vi "Table Test Sequencer.vi"(10 "Action":T1=enum."Run Position", 11 "Test Table":string[][](table)=[["1", "10mA", "10"], ["2", "20mA", "20"], ["3", "100mA", "10"], ["4", "20mA", "20"]]) -> (0 "Current Elapsed":dbl format="%.2g", 1 "CountDown Time":dbl format="%.2g", 2 "Test Running":bool, 3 "Current Test":string[](array[string]), 4 "Current Step ID":i32=-1, 5 "CountDown Pie":picture, 6 "Test Table Out":string[][](array[string])=[["1", "10mA", "1"], ["2", "20mA", "2"], ["3", "100mA", "1"], ["4", "20mA", "2"]], 7 "CountDown Text":string="0:00")   [LabVIEW 2018]
uses:
  Controls/StateMachineStates_TEST_TDEF.ctl
  Controls/Step Control Methods ENUM_TEST_TDef.ctl
  Controls/Timer Actions ENUM_TEST_TDef.ctl
  Controls/Stability State.ctl
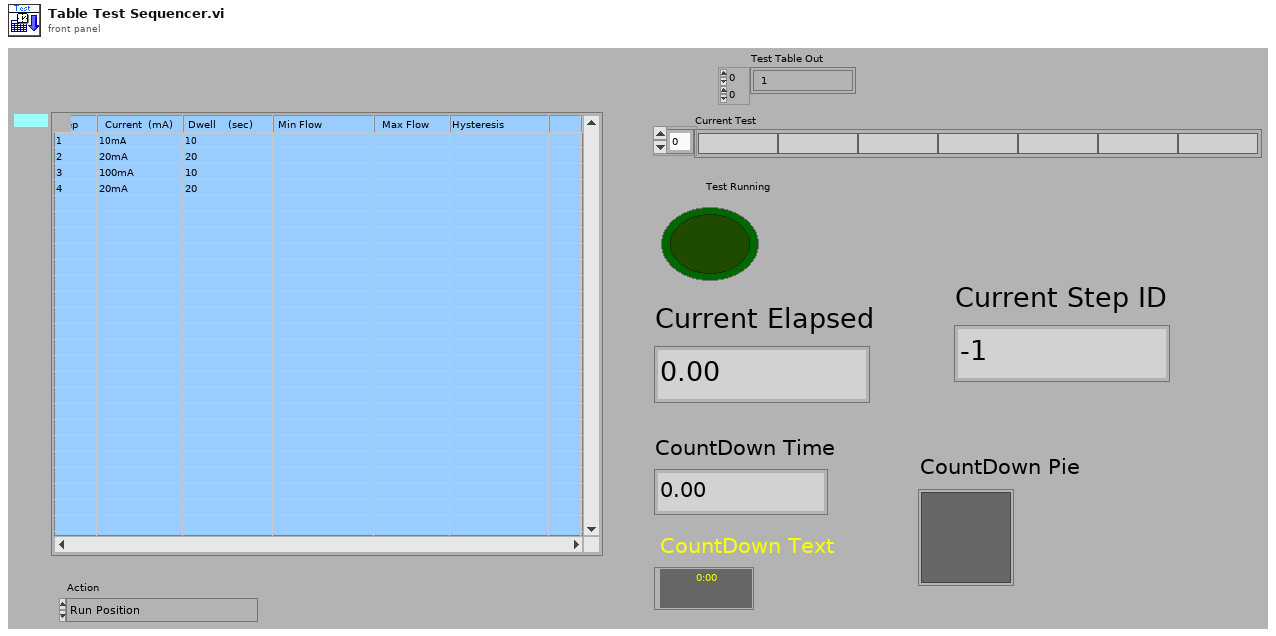
[diagram p1: front panel]
types:
  T1 = typedef "StateMachineStates_TEST_TDEF.ctl" = enum16{"Initialize", "Start", "Run Position", "Pause", "Resume", "Get Step", "Force Previous Step", "Force Next Step", "Stay on Current Step"}
  T2 = typedef "Stability State.ctl" = enum16{"Min Dwell Time", "Stability Dwell Time"}
  T3 = typedef "Timer Actions ENUM_TEST_TDef.ctl" = enum16{"Set Time", "Get Time", "Pause Time", "Resume Time"}
  T4 = typedef "Step Control Methods ENUM_TEST_TDef.ctl" = enum16{"Set Steps", "Get Current", "Goto Previous Step", "Goto Next Step", "Reset"}
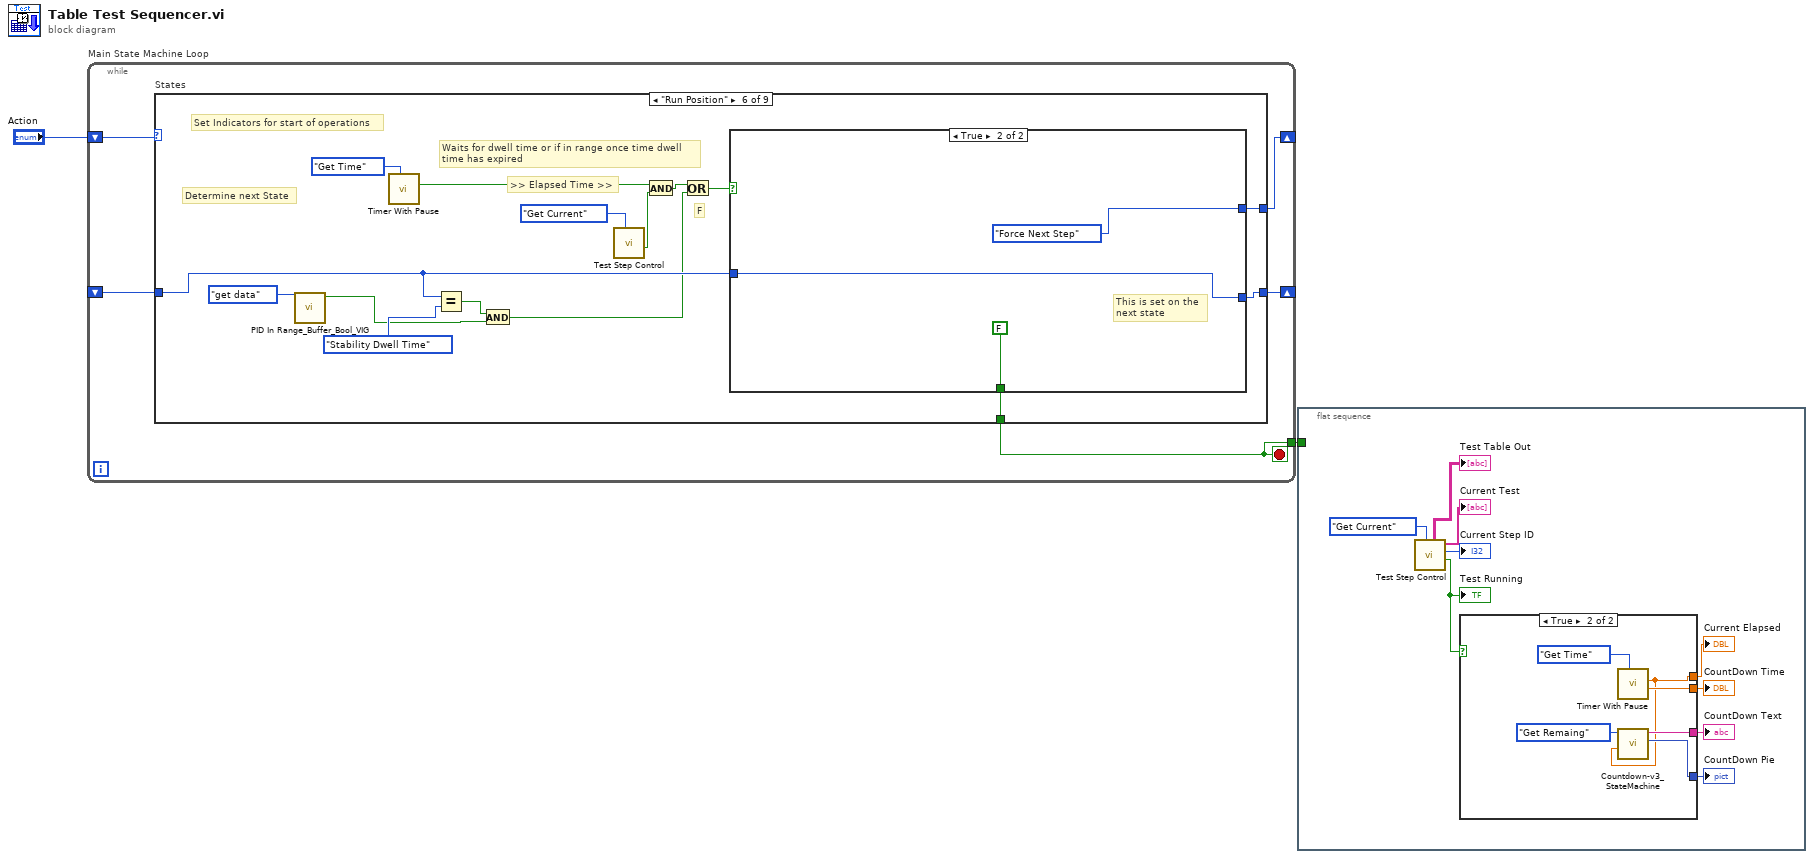
[diagram p0: block diagram]
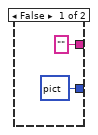
[diagram p2: hidden frame]
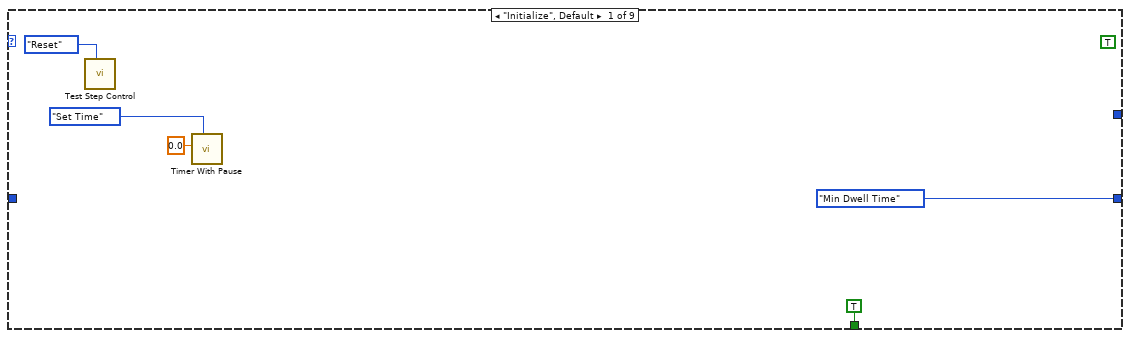
[diagram p3: hidden frame]
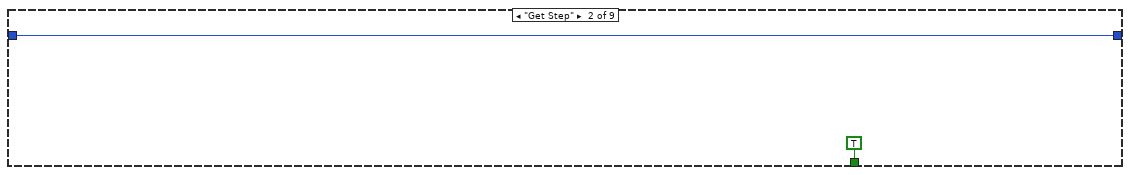
[diagram p4: hidden frame]
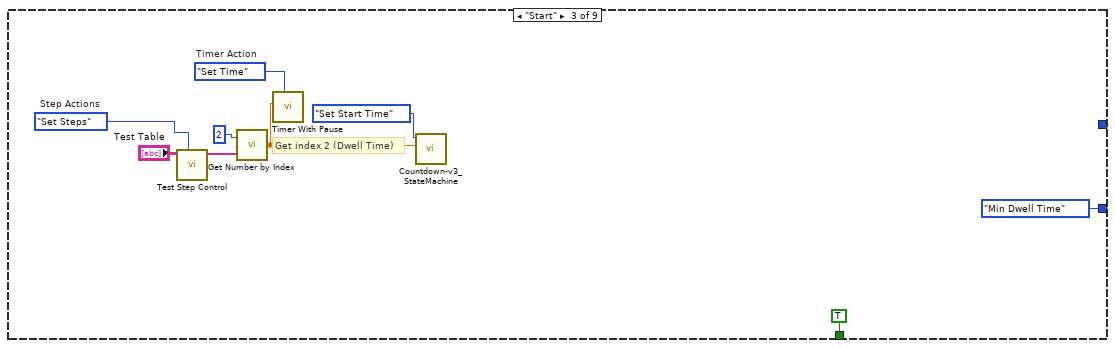
[diagram p5: hidden frame]
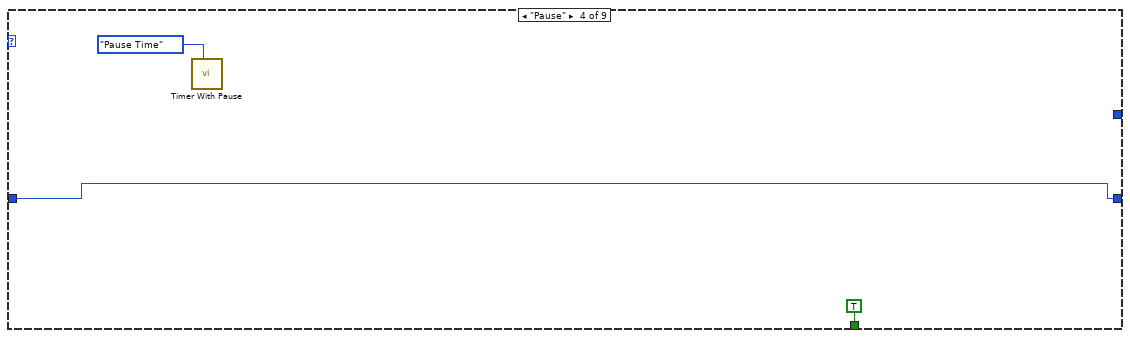
[diagram p6: hidden frame]
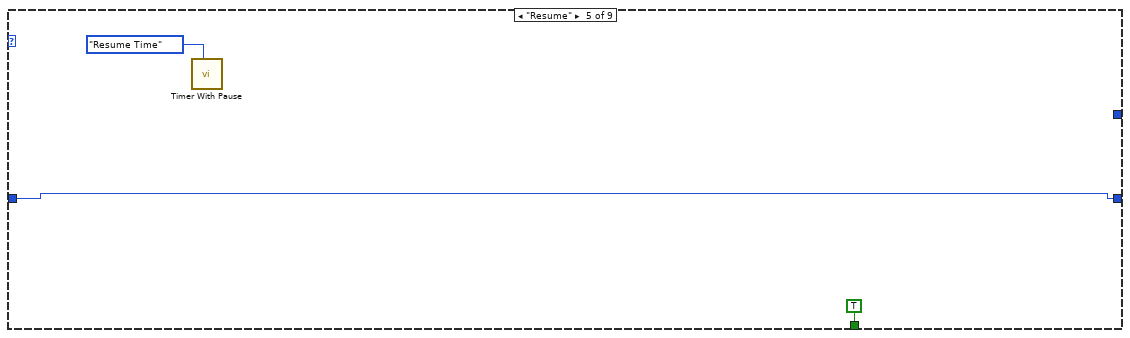
[diagram p7: hidden frame]
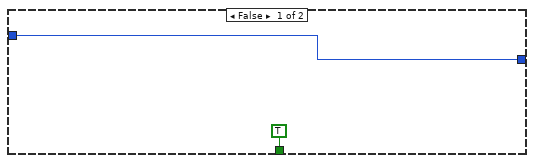
[diagram p8: hidden frame]
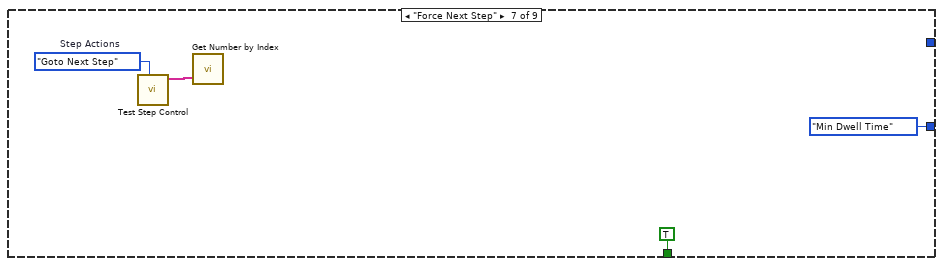
[diagram p9: hidden frame]
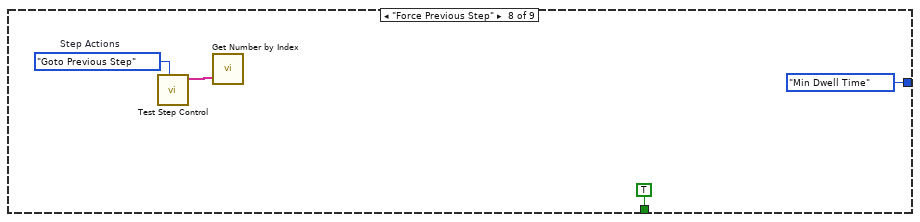
[diagram p10: hidden frame]
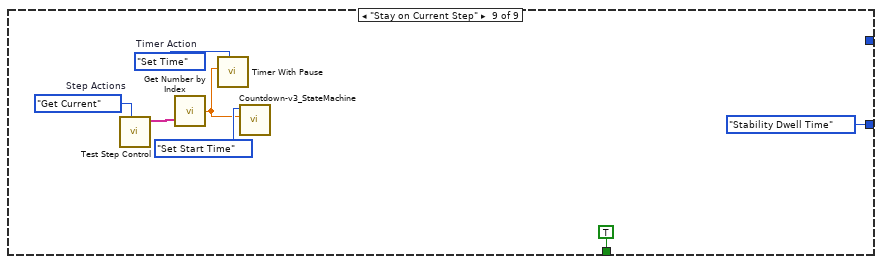
[diagram p11: hidden frame]
diagram:
  n1 = while "Main State Machine Loop" {
    tunnel: [w4] -> w2
    shift-right: [w7] -> _
    shift-left: _ -> [w6]
    shift-right: [w3] -> _
    shift-left: "Action" -> [w5]
    stop <- w4 stop-if-true
    n2 = case "States" shown="\"Run Position\"" w5 {
      tunnel: [Stability_State."Min Dwell Time" ("Enum") w14 Stability_State."Min Dwell Time" ("Enum") w25 w28 w43 Stability_State."Min Dwell Time" ("Enum") Stability_State."Min Dwell Time" ("Enum") Stability_State."Stability Dwell Time" ("Enum")] -> w7
      tunnel: w6 -> [_ w14 _ w25 w28 w35 _ _ _]
      tunnel: [TRUE TRUE TRUE TRUE TRUE w42 TRUE TRUE TRUE] -> w4
      tunnel: [_ _ _ _ _ w41 _ _ _] -> w3
      frame "Initialize", Default {
        (unwired) TRUE
        n3 = call "Test Step Control.vi"("Step Actions"=Step_Control_Methods_ENUM_TEST_TDef."Reset") -> ()  [unwired: 6 in, 5 out]
        n4 = call "Timer With Pause.vi"("Timer Action"=Timer_Actions_ENUM_TEST_TDef."Set Time", "Target Time"=0.0) -> ()  [unwired: 6 in, 4 out]
      }
      frame "Get Step" {
      }
      frame "Start" {
        w22 = Timer_Actions_ENUM_TEST_TDef."Set Time"  # Timer Action
        w23 = Step_Control_Methods_ENUM_TEST_TDef."Set Steps"  # Step Actions
        # "Get index 2 (Dwell Time)"
        n5 = call "Test Step Control.vi"("Step Actions"=w23, "Test Table"="Test Table") -> ("Current Test Step Parameters"=w21:string[])  [unwired: 5 in, 4 out]
        n6 = call "Get Number by Index.vi"("Test Table"=w21, "Index"=2) -> ("Dwell Time"=w17:dbl)
        n7 = call "Timer With Pause.vi"("Timer Action"=w22, "Target Time"=w17) -> ()  [unwired: 6 in, 4 out]
        n8 = call "Countdown-v3_StateMachine.vi"("Target Time"=w17, "Action"=enum16{"Set Start Time", "Get Remaing"}."Set Start Time") -> ()  [unwired: 8 in, 2 out]
      }
      frame "Pause" {
        n9 = call "Timer With Pause.vi"("Timer Action"=Timer_Actions_ENUM_TEST_TDef."Pause Time" ("t")) -> ()  [unwired: 7 in, 4 out]
      }
      frame "Resume" {
        n10 = call "Timer With Pause.vi"("Timer Action"=Timer_Actions_ENUM_TEST_TDef."Resume Time" ("t")) -> ()  [unwired: 7 in, 4 out]
      }
      frame "Run Position" {
        # "F"
        # "Waits for dwell time or if in range once time dwell\ntime has expired"
        # ">> Elapsed Time >>"
        # "Determine next State"
        # "Set Indicators for start of operations"
        n11 = call "PID In Range_Buffer_Bool_VIG.vi"("Operation"=enum16{"get data", "set data", "initialize"}."get data") -> ("Boolean 2"=w32:bool)  [unwired: 8 in, 2 out]
        n12 = call "Timer With Pause.vi"("Timer Action"=Timer_Actions_ENUM_TEST_TDef."Get Time") -> ("Done?"=w38:bool)  [unwired: 7 in, 3 out]
        n13 = Equal?(x=w35, y=Stability_State."Stability Dwell Time" ("Enum")) -> (x = y?=w33:bool)
        n14 = And(x=w33, y=w32) -> (x .and. y?=w31:bool)
        n15 = call "Test Step Control.vi"("Step Actions"=Step_Control_Methods_ENUM_TEST_TDef."Get Current") -> ("Test Running"=w40:bool)  [unwired: 6 in, 4 out]
        n16 = And(x=w38, y=w40) -> (x .and. y?=w44:bool)
        n17 = Or(x=w44, y=w31) -> (x .or. y?=w30:bool)
        n18 = case shown="True" w30 {
          tunnel: [w46 w47] -> w43
          tunnel: w35 -> [w46 w47]
          tunnel: [TRUE FALSE] -> w42
          tunnel: [_ StateMachineStates_TEST_TDEF."Force Next Step" ("f")] -> w41
          frame False {
          }
          frame True {
            # "This is set on the \nnext state"
          }
        }
      }
      frame "Force Next Step" {
        w52 = Step_Control_Methods_ENUM_TEST_TDef."Goto Next Step"  # Step Actions
        n19 = call "Test Step Control.vi"("Step Actions"=w52) -> ("Current Test Step Parameters"=w51:string[])  [unwired: 6 in, 4 out]
        n20 = call "Get Number by Index.vi"("Test Table"=w51) -> ()  [unwired: 1 in, 1 out]
      }
      frame "Force Previous Step" {
        w56 = Step_Control_Methods_ENUM_TEST_TDef."Goto Previous Step"  # Step Actions
        n21 = call "Test Step Control.vi"("Step Actions"=w56) -> ("Current Test Step Parameters"=w55:string[])  [unwired: 6 in, 4 out]
        n22 = call "Get Number by Index.vi"("Test Table"=w55) -> ()  [unwired: 1 in, 1 out]
      }
      frame "Stay on Current Step" {
        w62 = Timer_Actions_ENUM_TEST_TDef."Set Time"  # Timer Action
        w63 = Step_Control_Methods_ENUM_TEST_TDef."Get Current"  # Step Actions
        n23 = call "Test Step Control.vi"("Step Actions"=w63) -> ("Current Test Step Parameters"=w61:string[])  [unwired: 6 in, 4 out]
        n24 = call "Get Number by Index.vi"("Test Table"=w61) -> ("Dwell Time"=w59:dbl)  [unwired: 1 in]
        n25 = call "Timer With Pause.vi"("Timer Action"=w62, "Target Time"=w59) -> ()  [unwired: 6 in, 4 out]
        n26 = call "Countdown-v3_StateMachine.vi"("Target Time"=w59, "Action"=enum16{"Set Start Time", "Get Remaing"}."Set Start Time") -> ()  [unwired: 8 in, 2 out]
      }
    }
  }
  n27 = flat-sequence {
    tunnel: w2 -> [_]
    frame #0 {
      n28 = call "Test Step Control.vi"("Step Actions"=Step_Control_Methods_ENUM_TEST_TDef."Get Current") -> ("Test Running"=w70:bool, "Current Test Step Index"=→"Current Step ID":i32, "Current Test Step Parameters"=→"Current Test":string[], "Test Table Out"=→"Test Table Out":string[][])  [unwired: 6 in, 1 out]
      "Test Running" <- w70
      n29 = case shown="True" w70 {
        tunnel: [_ w76] -> w68
        tunnel: [_ w80] -> w69
        tunnel: ["" ("Remaining") w78] -> w66
        tunnel: [picture data[5B] ("new picture") w77] -> w65
        frame False {
        }
        frame True {
          n30 = call "Timer With Pause.vi"("Timer Action"=Timer_Actions_ENUM_TEST_TDef."Get Time") -> ("CountDown Time"=w80:dbl, "Elapsed Time"=w76:dbl)  [unwired: 7 in, 2 out]
          n31 = call "Countdown-v3_StateMachine.vi"("Elapsed Time"=w76, "Action"=enum16{"Set Start Time", "Get Remaing"}."Get Remaing") -> ("new picture"=w77:picture, "Remaining"=w78:string)  [unwired: 8 in]
        }
      }
      "Current Elapsed" <- w68
      "CountDown Time" <- w69
      "CountDown Text" <- w66
      "CountDown Pie" <- w65
    }
  }
